vi "Read Quadrature.vi"(8 "error in (no error)":errorcluster, 11 "SD Module in":refnum<class "SD Module.lvclass">) -> (0 "error out":errorcluster, 2 "Quadrature":T1 {"Quadrature Channels"."Index Mode" items=["Disabled", "Phase B0 A0", "Phase B0 A1", "Phase B1 A0", "Phase B1 A1"]; "Quadrature Channels"."Timebase" items=["256 us", "512 us", "1024 us", "2048 us", "4096 us", "8192 us", "16384 us", "32768 us"]}, 3 "SD Module out":refnum<class "SD Module.lvclass">)   [LabVIEW 2020, in "Modules.lvlib" / "SD Module.lvclass"]
uses:
  SD Module.lvclass
  Type Defs/Quadrature.ctl
  Type Defs/Quadrature Channel.ctl
  SD Module.lvclass/SD Module.ctl
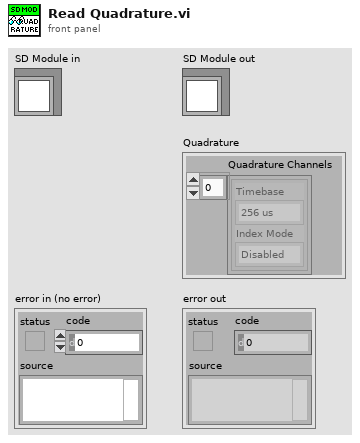
[diagram p1: front panel]
types:
  T1 = typedef "Modules.lvlib/SD Module.lvclass/Quadrature.ctl" = cluster{"Quadrature Channels":T2[]}
  T2 = typedef "Modules.lvlib/SD Module.lvclass/Quadrature Channel.ctl" = cluster{"Timebase":u32, "Index Mode":u32}
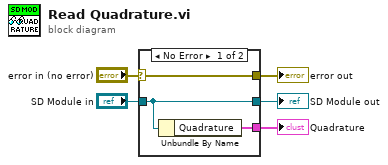
[diagram p0: block diagram]
diagram:
  n1 = case shown="No Error" "error in (no error)" {
    selector: "error in (no error)" -> [w8 w9]
    tunnel: [w8 w9] -> w4
    tunnel: [w7 w10] -> w2
    tunnel: "SD Module in" -> [w7 w10]
    tunnel: [w6 _] -> w1
    frame No Error {
      n2 = Unbundle By Name(w7) -> ("Quadrature"=w6:T1)
    }
    frame Error {
    }
  }
  "error out" <- w4
  "SD Module out" <- w2
  "Quadrature" <- w1
